vi "UiSchematic_b2g2.vi"() -> ()   [LabVIEW 2011]
uses:
  Regelventil.ctl
  Pumpe.ctl
  Ventil_Senkrecht.ctl
  Ventil_Waagrecht.ctl
  Output - Cluster b2g2.ctl
  <vilib>/Platform/TimedLoop/XDataNode/timing_clust.ctl
  <vilib>/Platform/TimedLoop/XDataNode/nitl_modes.ctl
  <vilib>/Platform/TimedLoop/XDataNode/wakeup.ctl
  <vilib>/Platform/TimedLoop/XDataNode/XDataNode.xnode
  <vilib>/Platform/TimedLoop/XDataNode/XDNodeRunTimeDep.lvlib
panel:
  out "target connection":bool
  out "T-2 Min!":bool
  out "T-2 Max!":bool
  out "V-14":T1
  out "V-33":T2
  out "V-34":T2
  out "V-35":T2
  out "V-10":T2
  out "P-4 [%]":u8
  out "P-4 ERR":bool
  out "P-4":T3
  out "DFS-1 [dl]":u64
  out "DFS-1 [l/min]":dbl format="%.2f"
  out "HS-1":bool
  out "TS-5 [°C]":dbl format="%.2g"
  out "pHS-1 [pH]":dbl format="%.2g"
  out "TS-4 [°C]":dbl format="%.2g"
  out "DS-1 [bar]":dbl format="%.2g"
  out "V-15":u8
  out "V-15":T4
  out "V-13":u8
  out "V-13":T4
  out "MR Min! 2":bool
  out "MR Max! 2":bool
  out "FS-2 [l]":dbl(slide) scale=10.0..80.0 scale format="%#.2g"
  out "FS-3 [l]":dbl(slide) scale=0.0..5.0 scale format="%#.1g"
  in  "stop":bool
  out "T-1 Min!":bool
  out "T-1 Max!":bool
  out "FS-1 [l]":dbl(slide) scale=10.0..80.0 scale format="%#.2g"
  # "B2G2"
  # "T-2"
  # "T-1"
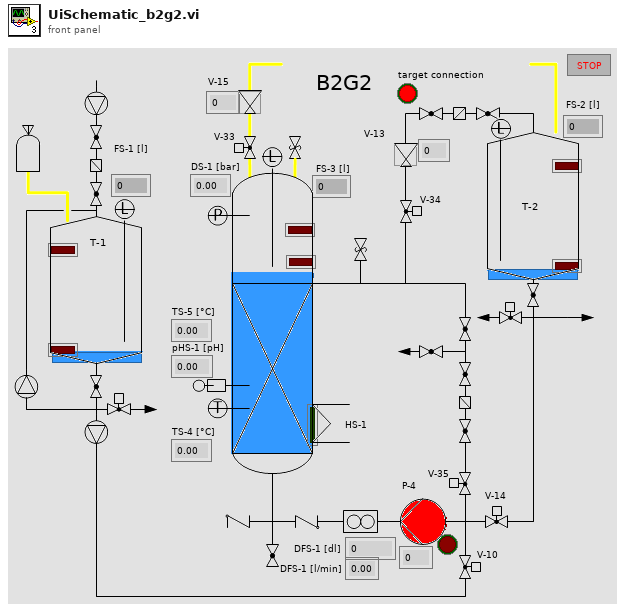
[diagram p1: front panel]
types:
  T1 = typedef "Ventil_Waagrecht.ctl" = u16
  T2 = typedef "Ventil_Senkrecht.ctl" = u16
  T3 = typedef "Pumpe.ctl" = bool
  T4 = typedef "Regelventil.ctl" = bool
  T5 = typedef "Output - Cluster b2g2.ctl" = cluster{"DFS-1 [dl]":u64, "FS-3 [l]":dbl, "DFS-1 [l/min]":dbl, "DS-1 [bar]":dbl, "V-10 ZU":bool, "V-14 ZU":bool, "FS-1 [l]":dbl, "FS-2 [l]":dbl, "TS-4 [°C]":dbl, "HS-1":bool, "V-13 [%]":u8, "V-15 [%]":u8, "P-4 [%]":u8, "Dosierung":bool, "MR Max Füllstand":bool, "MR Min Füllstand":bool, "Dosiermenge [l]":sgl, "V-14 AUF":bool, "V-10 AUF":bool, "T-1 Max Füllstand":bool, "T-1 Min Füllstand":bool, "T-2 Max Füllstand":bool, "T-2 Min Füllstand":bool, "pHS-1 [pH]":dbl, "P-4 RUN":bool, "V-33 AUF":bool, "V-33 ZU":bool, "V-34 AUF":bool, "V-34 ZU":bool, "P-4 ERR":bool, "TS-5 [°C]":dbl, "V-35 AUF":bool, "V-35 ZU":bool, "P-9 RUN":bool}
  T6 = typedef "XDNodeRunTimeDep.lvlib/timing_clust.ctl" = cluster{"Expected End [f-1]":u64, "Actual End [f-1]":u64, "Finished Late? [f-1]":bool, "Expected End [i-1]":u64, "Actual End [i-1]":u64, "Finished Late? [i-1]":bool, "Expected Start [i]":u64, "Actual Start [i]":u64, "Expected Start [f]":u64, "Actual Start [f]":u64, "Source Name":string, "Structure Name":string, "Period":i64, "Deadline":i64, "Offset":i64, "Start":i64, "Priority":i32, "Timeout":i32, "Mode":T7, "Wakeup Reason":T8, "Error":errorcluster, "Source Type":string, "Secondary Source Type":string, "Global End Time":u64, "Global Start Time":u64, "Frame Duration":u64, "Iteration Duration":u64, "Assigned CPU":i32, "I/O Scan Engine Mode":u32}
  T7 = typedef "XDNodeRunTimeDep.lvlib/nitl_modes.ctl" = enum32{"No Change", "Process missed periods, maintain original phase", "Discard missed periods, maintain original phase", "Process missed periods, ignore original phase", "Discard missed periods, ignore original phase"}
  T8 = typedef "XDNodeRunTimeDep.lvlib/wakeup.ctl" = enum32{"Normal", "Aborted", "Asynchronous wakeup", "Timing source error", "Timed loop error", "Timeout"}
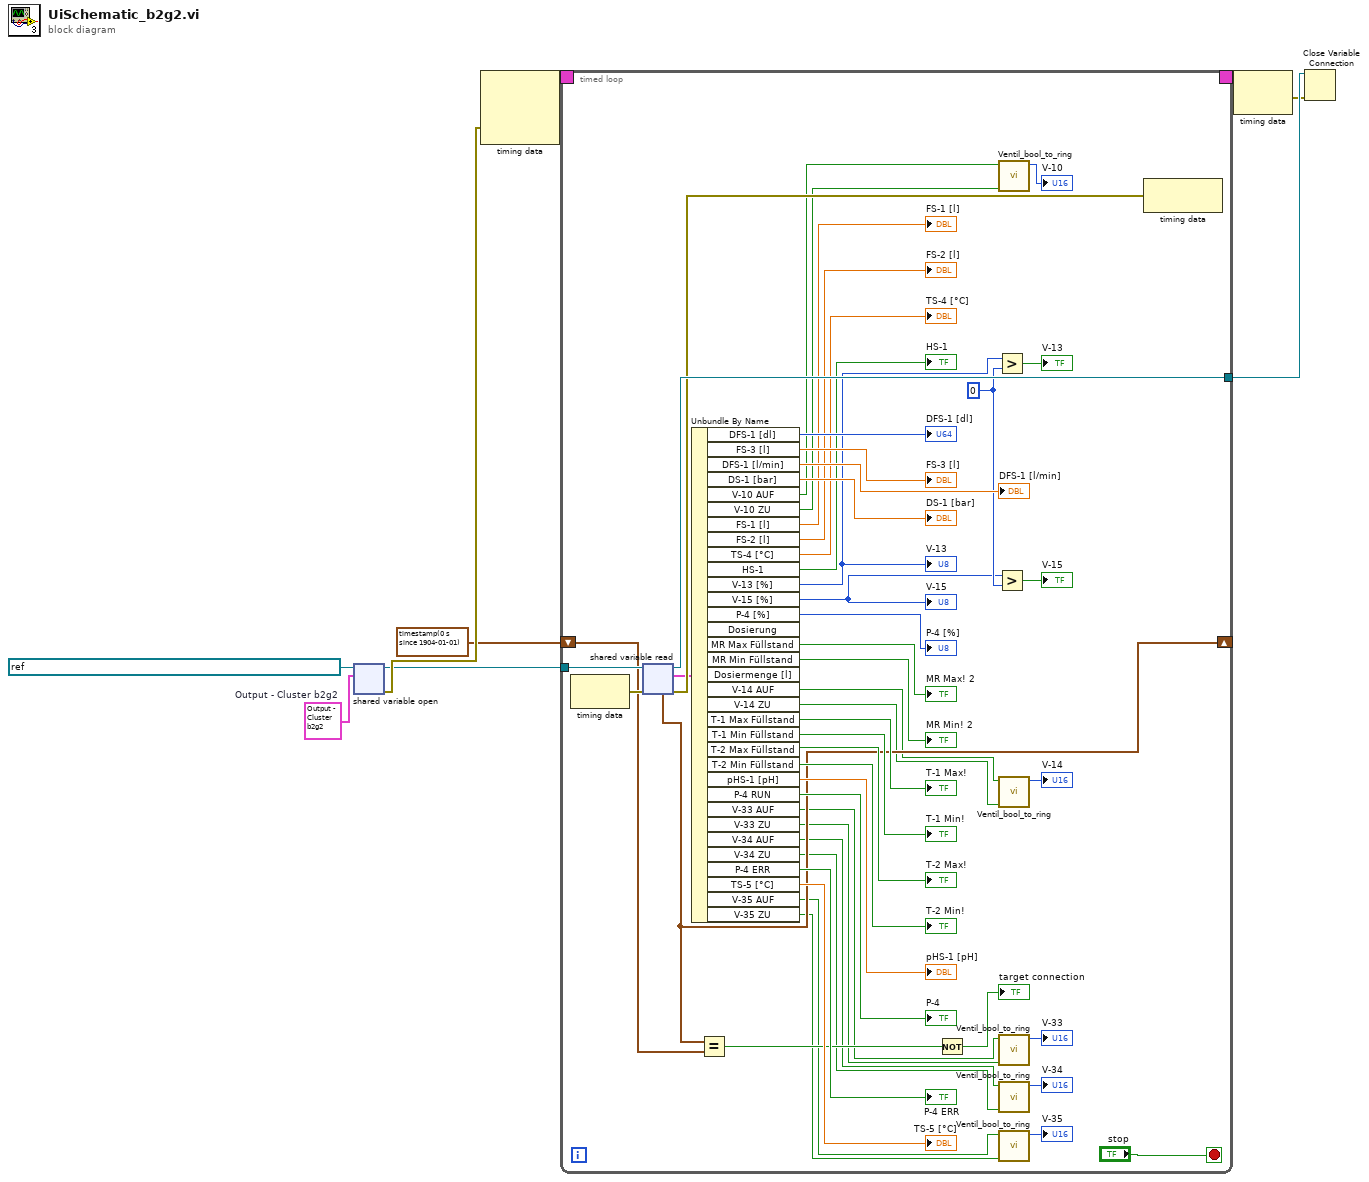
[diagram p0: block diagram]
diagram:
  w4 = T5 {"DFS-1 [dl]"=0, "FS-3 [l]"=0.0, "DFS-1 [l/min]"=0.0, "DS-1 [bar]"=0.0, "V-10 ZU"=FALSE, "V-14 ZU"=FALSE, "FS-1 [l]"=0.0, "FS-2 [l]"=0.0, "TS-4 [°C]"=0.0, "HS-1"=FALSE, "V-13 [%]"=0, "V-15 [%]"=0, "P-4 [%]"=0, "Dosierung"=FALSE, "MR Max Füllstand"=FALSE, "MR Min Füllstand"=FALSE, "Dosiermenge [l]"=0.0, "V-14 AUF"=FALSE, "V-10 AUF"=FALSE, "T-1 Max Füllstand"=FALSE, "T-1 Min Füllstand"=FALSE, "T-2 Max Füllstand"=FALSE, "T-2 Min Füllstand"=FALSE, "pHS-1 [pH]"=0.0, "P-4 RUN"=FALSE, "V-33 AUF"=FALSE, "V-33 ZU"=FALSE, "V-34 AUF"=FALSE, "V-34 ZU"=FALSE, "P-4 ERR"=FALSE, "TS-5 [°C]"=0.0, "V-35 AUF"=FALSE, "V-35 ZU"=FALSE, "P-9 RUN"=FALSE}  # Output - Cluster b2g2
  n1 = shared-variable-open(refnum<k21> "ni.var.psp://10.27.40.25/variables - b2g2/data - network b2g2" ("Output Var B2G2"), w4) -> (w3:refnum<k21>, w6:errorcluster)  [unwired: 2 in]
  n2 = node-c288(w6) -> (w9:T6)  [unwired: 2 in]
  n3 = timed-loop {
    timing: w9 -> [_]
    timing-out: [_] -> w8
    tunnel: [w58] -> w7
    tunnel: w3 -> [w57]
    shift-right: [w27] -> _
    shift-left: timestamp(0 s since 1904-01-01) -> [w28]
    stop <- "stop" stop-if-true
    w40 = u8 0 ("y")
    n4 = node-c288() -> (w56:errorcluster)  [unwired: 1 in]
    n5 = shared-variable-read(w57, w56) -> (w58:refnum<k21>, w55:errorcluster, w54:T5, w27:timestamp)
    n6 = Unbundle By Name(w54) -> ("DFS-1 [dl]"=→"DFS-1 [dl]":u64, "FS-3 [l]"=→"FS-3 [l]":dbl, "DFS-1 [l/min]"=→"DFS-1 [l/min]":dbl, "DS-1 [bar]"=→"DS-1 [bar]":dbl, "V-10 AUF"=w21:bool, "V-10 ZU"=w13:bool, "FS-1 [l]"=→"FS-1 [l]":dbl, "FS-2 [l]"=→"FS-2 [l]":dbl, "TS-4 [°C]"=→"TS-4 [°C]":dbl, "HS-1"=→"HS-1":bool, "V-13 [%]"=w33:u8, "V-15 [%]"=w39:u8, "P-4 [%]"=→"P-4 [%]":u8, "MR Max Füllstand"=→"MR Max! 2":bool, "MR Min Füllstand"=→"MR Min! 2":bool, "V-14 AUF"=w23:bool, "V-14 ZU"=w14:bool, "T-1 Max Füllstand"=→"T-1 Max!":bool, "T-1 Min Füllstand"=→"T-1 Min!":bool, "T-2 Max Füllstand"=→"T-2 Max!":bool, "T-2 Min Füllstand"=→"T-2 Min!":bool, "pHS-1 [pH]"=→"pHS-1 [pH]":dbl, "P-4 RUN"=→"P-4":bool, "V-33 AUF"=w18:bool, "V-33 ZU"=w12:bool, "V-34 AUF"=w17:bool, "V-34 ZU"=w11:bool, "P-4 ERR"=→"P-4 ERR":bool, "TS-5 [°C]"=→"TS-5 [°C]":dbl, "V-35 AUF"=w16:bool, "V-35 ZU"=w10:bool)  [unwired: 2 out]
    "V-15" <- w39
    "V-13" <- w33
    n7 = Equal?(x=w27, y=w28) -> (x = y?=w25:bool)
    n8 = Not(x=w25) -> (.not. x?=→"target connection":bool)
    n9 = Greater?(x=w33, y=w40) -> (0:→"V-13":bool)
    n10 = Greater?(x=w39, y=w40) -> (0:→"V-15":bool)
    n11 = call "Ventil_bool_to_ring.vi"("ZU"=w13, "AUF"=w21) -> ("ring"=→"V-10":i32)  [unwired: 9 in]
    n12 = call "Ventil_bool_to_ring.vi"("ZU"=w14, "AUF"=w23) -> ("ring"=→"V-14":i32)  [unwired: 9 in]
    n13 = call "Ventil_bool_to_ring.vi"("ZU"=w12, "AUF"=w18) -> ("ring"=→"V-33":i32)  [unwired: 9 in]
    n14 = call "Ventil_bool_to_ring.vi"("ZU"=w11, "AUF"=w17) -> ("ring"=→"V-34":i32)  [unwired: 9 in]
    n15 = call "Ventil_bool_to_ring.vi"("ZU"=w10, "AUF"=w16) -> ("ring"=→"V-35":i32)  [unwired: 9 in]
    n16 = node-c288(w55) -> ()  [unwired: 1 out]
  }
  n17 = node-c288(w8) -> (w2:errorcluster)
  n18 = Close Variable Connection(8:w2, 11:w7) -> ()  [unwired: 1 out]
